vi "E11111.vi"(8 "error in (no error)":errorcluster, 11 "Signal":waveform(dbl)) -> (0 "error out":errorcluster)   [LabVIEW 2022 SP3, in "Demo.lvlib" / "E11111.lvclass"]
uses:
  E11111.lvclass
  C:/Users/jakub/repos/gh/lv-error/Source/Error/Error/Error.lvclass
  E11111.lvclass/E11111.ctl
  Error/Error/Error.lvclass
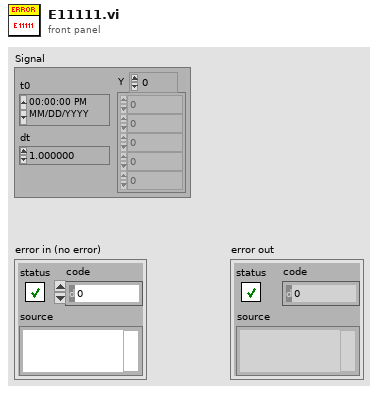
[diagram p1: front panel]
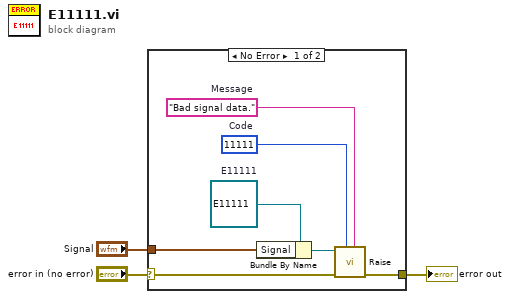
[diagram p0: block diagram]
diagram:
  n1 = case shown="No Error" "error in (no error)" {
    selector: "error in (no error)" -> [w10 w11]
    tunnel: [w9 w11] -> w2
    tunnel: "Signal" -> [w7 _]
    frame No Error {
      w4 = "Bad signal data."  # Message
      w5 = 11111  # Code
      w8 = refnum<class "E11111.lvclass"> refnum  # E11111
      n2 = Bundle By Name(cluster=w8, "Signal"=w7) -> (w6:refnum<class "E11111.lvclass">)
      n3 = call "Raise.vi"("Message"=w4, "Code"=w5, "error in (no error)"=w10, "Error in"=w6) -> ("error out"=w9:errorcluster)  [unwired: 6 in, 1 out]
    }
    frame Error {
    }
  }
  "error out" <- w2
